vi "Set Or Get Value.vi"(7 "Signal":bool, 8 "error in (no error)":errorcluster caption="错误输入（无错误）", 9 "Mode":T1, 11 "Table Ref In":refnum<vi>) -> (0 "error out":errorcluster caption="错误输出", 3 "Table Ref Out":refnum<vi>)   [LabVIEW 2012, in "Table Tool.lvlib"]
uses:
  Table Tool.lvlib
  GetOrSet.ctl
panel:
  in  "Value In":string[][](array[string])
  out "Value Out":string[][](array[string])
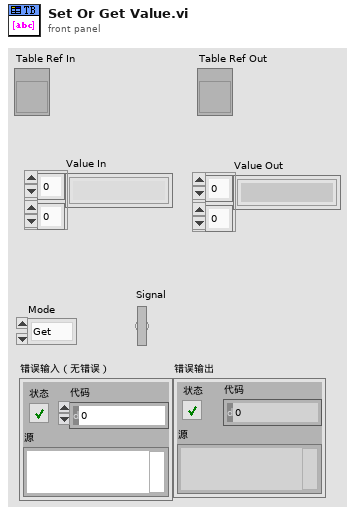
[diagram p1: front panel]
types:
  T1 = typedef "Table Tool.lvlib/GetOrSet.ctl" = enum16{"Get", "Set"}
  T2 = typedef "LVRowAndColumnTypeDef.ctl" = cluster{"Row":i32, "Column":i32}
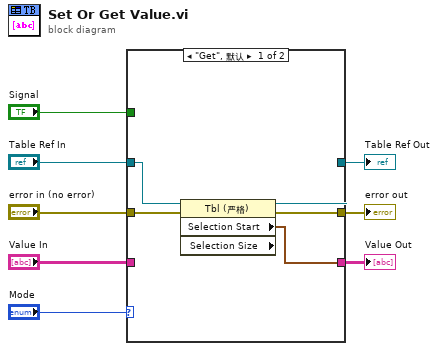
[diagram p0: block diagram]
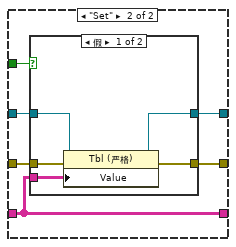
[diagram p2: hidden frame]
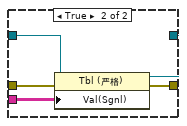
[diagram p3: hidden frame]
diagram:
  n1 = case shown="\"Get\", 默认" "Mode" {
    tunnel: "Table Ref In" -> [w12 w18]
    tunnel: "error in (no error)" -> [w13 w19]
    tunnel: [w10 w16] -> w5
    tunnel: [w11 w17] -> w4
    tunnel: "Value In" -> [_ w15]
    tunnel: [w9 w15] -> w3
    tunnel: "Signal" -> [_ w14]
    frame "Get", Default {
      n2 = property class="Tbl (严格)" props=["Selection Start", "Selection Size"](reference=w12, error in=w13) -> (reference out=w11:refnum<vi>, error out=w10:errorcluster, "Selection Start"=w9:T2)  [unwired: 1 out]
    }
    frame "Set" {
      n3 = case shown="假" w14 {
        tunnel: w19 -> [w23 w29]
        tunnel: w18 -> [w24 w28]
        tunnel: [w20 w27] -> w17
        tunnel: [w21 w26] -> w16
        tunnel: w15 -> [w22 w25]
        frame False {
          n4 = property class="Tbl (严格)"(reference=w24, error in=w23, "Value"=w22) -> (reference out=w20:refnum<vi>, error out=w21:errorcluster)
        }
        frame True {
          n5 = property class="Tbl (严格)"(reference=w28, error in=w29, "Val(Sgnl)"=w25) -> (reference out=w27:refnum<vi>, error out=w26:errorcluster)
        }
      }
    }
  }
  "Table Ref Out" <- w4
  "error out" <- w5
  "Value Out" <- w3
